vi "ReadIntakeEncoder.vi"() -> ()   [LabVIEW 2015]
uses:
  Common Code/Encoder Values Super Cluster.ctl
  Common Code/Encoder Values.ctl
  Robot Global Data.vi
panel:
  out "Quick Use Cluster":T1
  in  "Encoder Values Super Cluster":T1
  in  "Reset?":bool=TRUE
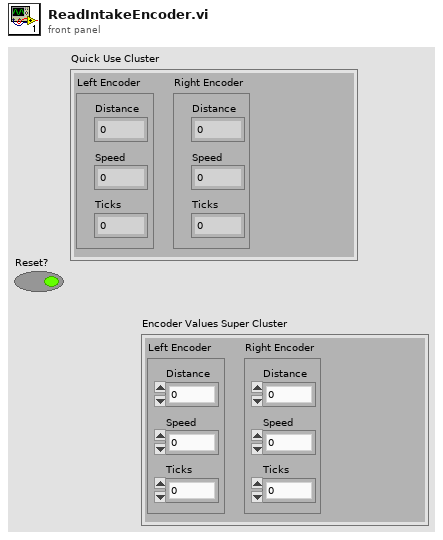
[diagram p1: front panel]
types:
  T1 = typedef "Encoder Values Super Cluster.ctl" = cluster{"Left Encoder":T2, "Right Encoder":T2}
  T2 = typedef "Encoder Values.ctl" = cluster{"Distance":dbl, "Speed":dbl, "Ticks":dbl}
  T3 = typedef "Dashboard Control Data.ctl" = cluster{"Auton Loops":dbl, "Shooter Presets":T4, "Encoder Control":T6, "Steer PID output":cluster{"output high":dbl, "output low":dbl}, " Steer PID gains":cluster{"proportional gain (Kc)":dbl, "integral time (Ti, min)":dbl, "derivative time (Td, min)":dbl}, "Drivetrain Settings":T7, "Vision Packet":T8, "Dashboard Drivetrain Command":T9, "Intake Command Cluster":T11}
  T4 = typedef "Shooter Presets.ctl" = cluster{"Batter Shot":T5, "Low Bar Curve Shot":T5, "Deep Middle Shot":T5, "Manual Shot":T5, "Left Ticks Per Rotation":dbl, "Right Ticks Per Rotation":dbl, "Low Bar Shot":T5, "Shooter RPM Tolerance":dbl, "IIR Filter Power":dbl, "Trigger Power":dbl}
  T5 = typedef "Shot Presets.ctl" = cluster{"Left Wheel RPM":dbl, "Right Wheel RPM":dbl}
  T6 = typedef "Encoder Control.ctl" = cluster{"Right Tick Constant":dbl, "Left Tick Constant":dbl, "Reset?":bool, "Y Dist":cluster{"PID gains":cluster{"proportional gain (Kc)":dbl, "integral time (Ti, min)":dbl, "derivative time (Td, min)":dbl}}, "Y Stop Thresh":dbl, "Y Stop Speed":dbl}
  T7 = typedef "Drivetrain Settings.ctl" = cluster{"Gyro Tolerance":dbl, "Throttle Ramp (ms)":dbl, "Angular rate compensation":bool, "Throttle to Rate Scale":dbl, "Rate compensation gain":dbl}
  T8 = typedef "Vision Packet.ctl" = cluster{"Distance":dbl, "Center X":dbl, "Center Y":dbl, "Found Target?":bool}
  T9 = typedef "Dashboard Drivetrain Command.ctl" = cluster{"Drivetrain Vision":T10, "Vision Scale Down Speed":dbl, "Vision PID gains":cluster{"proportional gain (Kc)":dbl, "integral time (Ti, min)":dbl, "derivative time (Td, min)":dbl}}
  T10 = typedef "Drivetrain Vision.ctl" = cluster{"High parameters":dbl, "Low parameters":dbl}
  T11 = typedef "Intake Command Cluster.ctl" = cluster{"Suck Speed":dbl, "Spit Speed":dbl, "Right Pot 0":dbl, "Left Pot 0":dbl, "Trigger Power":dbl, "Raise Speed":dbl, "Lower Speed":dbl}
  T12 = typedef "WPI_EncoderDevRef.ctl" = cluster{"DevStatus":errorcluster, "EncoderIndex":T13, "CounterIndex":T14, "DistancePerCount":dbl, "Decoding Type":T15}
  T13 = typedef "FPGA_EncoderIdx.ctl" = enum8{"Enc 0", "Enc 1", "Enc 2", "Enc 3", "Enc 4", "Enc 5", "Enc 6", "Enc 7", "Invalid"}
  T14 = typedef "FPGA_CounterCtrSystemIndex.ctl" = enum8{"Ctr 0", "Ctr 1", "Ctr 2", "Ctr 3", "Ctr 4", "Ctr 5", "Ctr 6", "Ctr 7", "Invalid"}
  T15 = typedef "WPI_EncoderType.ctl" = enum16{"1x", "2x", "4x"}
  T16 = cluster{"Ticks":dbl, "Distance":dbl, "Speed":dbl}
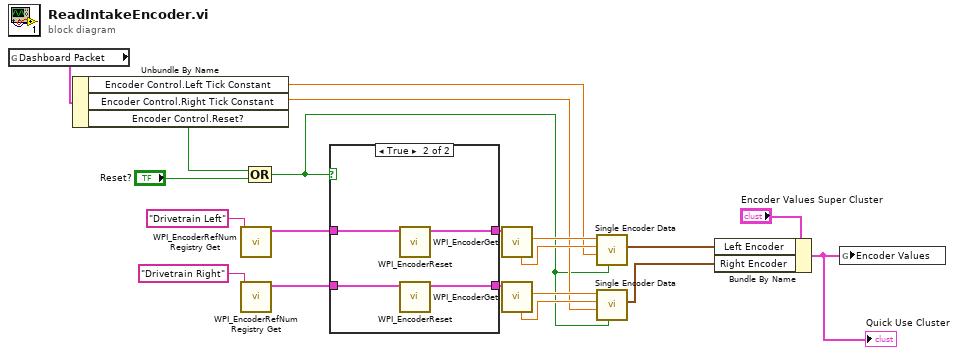
[diagram p0: block diagram]
diagram:
  n1 = global read "Robot Global Data.vi" "Dashboard Packet"() -> (w6:T3)
  n2 = Unbundle By Name(w6) -> ("Encoder Control.Left Tick Constant"=w3:dbl, "Encoder Control.Right Tick Constant"=w2:dbl, "Encoder Control.Reset?"=w5:bool)
  n3 = call <vilib>:"WPI_EncoderRefNum Registry Get.vi"("refnum name"="Drivetrain Left") -> ("EncoderDevRef"=w17:T12)  [unwired: 9 in, 1 out]
  n4 = call <vilib>:"WPI_EncoderRefNum Registry Get.vi"("refnum name"="Drivetrain Right") -> ("EncoderDevRef"=w18:T12)  [unwired: 9 in, 1 out]
  n5 = Compound Arithmetic op=OR(w5, "Reset?") -> (w1:bool)
  n6 = case shown="True" w1 {
    tunnel: w18 -> [w21 w25]
    tunnel: w17 -> [w22 w26]
    tunnel: [w22 w23] -> w16
    tunnel: [w21 w24] -> w15
    frame False {
    }
    frame True {
      n7 = call <vilib>:"WPI_EncoderReset.vi"("EncoderDevRef"=w26) -> ("EncoderDevRef"=w23:T12)  [unwired: 9 in, 1 out]
      n8 = call <vilib>:"WPI_EncoderReset.vi"("EncoderDevRef"=w25) -> ("EncoderDevRef"=w24:T12)  [unwired: 9 in, 1 out]
    }
  }
  n9 = call <vilib>:"WPI_EncoderGet.vi"("EncoderDevRef"=w16) -> ("Distance"=w14:dbl, "Rate"=w13:dbl)  [unwired: 5 in, 4 out]
  n10 = call <vilib>:"WPI_EncoderGet.vi"("EncoderDevRef"=w15) -> ("Distance"=w12:dbl, "Rate"=w11:dbl)  [unwired: 5 in, 4 out]
  n11 = call "Single Encoder Data.vi"("Reset?"=w1, "Tick Constant"=w3, "Rate"=w13, "Distance"=w14) -> ("output cluster"=w9:T16)  [unwired: 7 in]
  n12 = call "Single Encoder Data.vi"("Reset?"=w1, "Tick Constant"=w2, "Rate"=w11, "Distance"=w12) -> ("output cluster"=w8:T16)  [unwired: 7 in]
  n13 = Bundle By Name(cluster="Encoder Values Super Cluster", "Left Encoder"=w9, "Right Encoder"=w8) -> (w7:T1)
  "Quick Use Cluster" <- w7
  n14 = global write "Robot Global Data.vi" "Encoder Values"(w7) -> ()
